vi "Common substrings.vi"(8 "minimum pattern length(3)":i32=3, 9 "Include zero transitions (t)":bool=TRUE, 11 "Full transition sequence from service to end":string[](array[string])=["-2 0 3 0 -3 0 4 -4 0\r\n", "0 3\r\n", "0 4 -3 0 -4 1 0 4 -3 0\r\n", "0\r\n", "-2 0 3 -3 0 -4 1 -4 0 3 -3 4 -3 0 2 0 3\r\n", "0 3 0 1\r\n", "0 1 0 3\r\n", "0 3 -2 0 4\r\n", "0\r\n", "0 -3 4 0 2 -2 0 -3 0 3 -2 3 -3 4\r\n", "0 -3 4 -3 0\r\n", "-2 0 -2 2 0\r\n", "0 3 -2\r\n", "0 4 -3 0 3 -2 0 -3 4 -3 0 3 -2 2 -2 0 4 0\r\n", "2 0 1 -4 0 3 0 -4 4 0 -4 4 0 2 0 4 0 -3 4 -3 0 -4 0 4\r\n", "0 4\r\n", "-2 0 -2 0 3 0\r\n", "0 3 0 -2 3\r\n", "0 4 0 4 -4 0 2 0 -4 4 -3 0 -2 2 -2 0 4 -3 0 2 0 3 0\r\n", "0 4 -3 0 1 -1 0 3 0 -2 2 -2 0 -3 4 -3 0 4 -4 1 0\r\n", "", "0 -3\r\n", "2 0 3 0 1 0 -2 3\r\n", "0\r\n", "1 -1 0\r\n", "0 -2 3 0\r\n", "0 1 0 4 0 4 -4 4\r\n", "0 1 -1 0 3\r\n", "0 2 -2 3 -3 4\r\n", "-2 2 0 -2 3\r\n", "0 -1\r\n", "0 4 -4 4 0 3 0 -2 0 -4 0 1 -4\r\n", "-2 0 4 0 -3 3 0 -2 2 -2 0 -4 0 4 0\r\n", "0 -1 0 -4 4 -4 1 -4 0\r\n", "1 -4 1 0 2 0 -3 0 2 0 -2 0 1 0 1 -4 4 -4 1 0 3 -2 0 -4 4 -4\r\n", "0 1 -4 4 -4 1\r\n", "0 3 0 -3 3 0 1 0 1 -4 4\r\n", "0 1 -4 0 1 -4\r\n", "0 3 -2 0 1 -4 1 0 2 0 4 0 4 0 -1 2 -1 0\r\n", "1 0 -1 0 2 0 4 -4\r\n", "-4\r\n", "-1 0 4\r\n", "0 1 -1 0 1 -4 0\r\n", "-1 0 1 -4 0 3 0 2 0 4 0 -4 4 -4 0 -1 0 -4 0 -2 0 4\r\n", "0 4 0\r\n", "0 4 -4 0 2 -1 0 2 0 4 -4 1 -4 4 0 3\r\n", "0 4 0 2 0\r\n", "1 0 -1 1 0 -4 1 -4 1 0 -4\r\n", "0 3 -2 0 -4\r\n", "2 -1 0 -4 4 -4 0 2 0 4\r\n", "1 0\r\n", "-1 0 -1 1 0 -4\r\n", "0 3 0\r\n", "0 -4 4 -4 0 -4 0 4 0 2 0 1 -4 4\r\n", "-1 0 1 -4\r\n", "-1 0 2 -1 0 2\r\n", "1 -1 0 4 -4 1\r\n", "-1 0 1 -4 4 -4 0 -4 4\r\n", "0 3 0 3 0 1 -1 0 1\r\n", "-1 0 4 0 4 -4 1 0 -4 0\r\n", "1 0 4\r\n", "0 -1 0 2 -1 0 -2 3 -2 0 -4 4 -4\r\n", "0 3 0\r\n", "2 -1 0 1 -4 4 -4 0 2 0\r\n", "0 4 -4 1 0 1 0 1 -4 0 2 0 4 0 4 -4 1\r\n", "1 -1 0 3 0 3 0 1 0 4\r\n", "0 -4 0 -2 0 -4\r\n", "0 -4 4 -4 0 -2 0 2 0\r\n", "-1 0 4 -4 0\r\n", "1 0 -1 2 0 4\r\n", "0 2 0 -2 0\r\n", "0 1 -4 0 -4 0 3 -2 0 -4 0 -4 4 -4 1\r\n", "0 4 0 4 0 4 0 4 0 -2 3 0 3 0 4 0\r\n", "-4 -1\r\n", "-2 0 1 0 -4 4\r\n", "0 4\r\n", "-2 2 0 -1 -4 1 0 3 0\r\n", "-1 0 -1 2\r\n", "0 -1 1 0 4 0 3 -2 0 -2 3 -2 0 4 0 -2 2\r\n", "2 -1 0 4\r\n", "0 4 0 2 0 -2 0\r\n", "1 -1 0 3 0 -4 4 -4 0\r\n", "2 -1 0 3 -2 0 -3 0 3 0 -3 0\r\n", "0 4 0 4 -4 1 -1 0 -3 0 1 -4 1 0 4 0 -4 0 -4 4 -4 1\r\n", "0 -4 1 0 -4 4\r\n", "0 4 0 -2 2 -2 2 -2 2\r\n", "-2 2 -1 0 4 0 2 0 4 0 2 -2 0 4\r\n", "1 0 -1 0 -1 0 1 -1\r\n", "-2 2 -2 3\r\n", "1 0 -1 0 -1 2 0 2 -2 0 -4 0\r\n", "-2 2 0 3 -2 2\r\n", "0\r\n", "1 -1 0 3\r\n", "0 4 0\r\n", "-2 0 1 -4 0 -3 0\r\n", "1 0 -1 2 -1 1 -4\r\n", "0 4\r\n", "-2 0 -1 1\r\n", "0 3 0 3 0 3 -2\r\n", "-4 0 -4 4\r\n", "0 4 0 -4 0 -4\r\n", "-2 2 0 4 -4 0 2 -2\r\n", "-2 2 -2 0 -1\r\n", "0 4 -3 0\r\n", "0 1 0 -1 1\r\n", "-4 0\r\n", "-2 0 3 0 1 0 3 -2 0 -1 0 4 0 3 0 -3 3 -3\r\n", "0 4 0 -2 0 1 0 -4 4 -3 0 1 0 4 0 -4 1 0 3 -3 0\r\n", "0 -1 2\r\n", "2 0 -3 4 0\r\n", "-4 0 -3 3 -3 0 -3 3 0 -2 3 0\r\n", "0 -1 1 -4 4 -3 0 3 0\r\n", "0 -1 2 0 3 0 1 -4 4 0 2 0\r\n", "2 -2 0 -4 0 -4 4 0 -4\r\n", "1 -1 2 -1\r\n", "2 0 -2 0 4 0 2 0 3 0 -2 0 -4\r\n", "1 -1 0 -1\r\n", "0 1 -4 1\r\n", "0 4 0 -1 1 -1 0\r\n", "0 3\r\n", "-2 0\r\n", "1 -4 0 -2 0 4 0 -4 0 4 -3 0 1 -4 0 1\r\n", "0 -3 3 -2 0 3 0 -2 2\r\n", "1 0\r\n", "2\r\n", "0 -4\r\n", "0 4 0 -4 0 -3 3 -3 0 -2 0 -2 0 4 0 -1 1 0 3 0 -4 1 -4 0 4\r\n", "2 0 -1 1\r\n", "0 2 0 4 0 4 -4 0 -1 2\r\n", "0 3 -2 0 3 -2\r\n", "1 0 -3 3 0 -4\r\n", "0 -3 3 0 -1 0\r\n", "2 -2 0 1\r\n", "-4 1 -4 1 -4 0\r\n", "0 4 0 2 0 -4 1 2 -1 0 4 0 1 0 4 -4 4 0 -4 4 0\r\n", "-2 0 3 0 -2 0\r\n", "-2 2 -1 0 1 -4 0 3 -2\r\n", "1 -1 0 4 0 2 -2 3 0 1 -4 1 0 -3 4 0 3 0 4 0 4 0 -4 0\r\n", "-1 0 4 -4\r\n", "-1 0 -1 2 0 2 0\r\n", "-1 0 3 -2 0 2 -2 3 -2 2 -2 0 -3 4 0 1\r\n", "-2 2 -1 0 2 0 3 -1 3 -2 2 0 -2 2 -2 0 1 0 2 0\r\n", "1 -4 1 0 4 -4 0 2 0\r\n", "2 -2 0\r\n", "0 4 -4 -1 0 -1 1 -1 0 4 0 -2 3 -2 0\r\n", "-1 0 2 -1 0 4 -4 0 -4 0 4 0\r\n", "0 -3 0\r\n", "1 0 -1 2 -1 0 3 0 3 -2 3 -2 0 2\r\n", "2 0 2 0 -2 3 -2 2 -1 0 4 0 2\r\n", "-1 1 -4 1 0 1 0 -4 4 -4 0 3 -2 2 -1 0 3 0 -1 1\r\n", "2 0 -1 1 -1 0 3 -2 3 0 2 0 3 -2 0 -4 0 4 -4 0 4 0\r\n", "0 -1 0 3 0 2 -2\r\n", "1 -4 1 -1 0 2 0 3 -2 3 -2 3\r\n", "2 0\r\n", "-1 0 3 0 3\r\n", "1 -4 1 0 -4 4 -4 0\r\n", "-2 2 -1 0\r\n", "0 1 0 4 0 3 0 -2 0 3 0 4 0 2 -2 0\r\n", "0 3 -2 0 4 0 -2 2 -2 0 -2 0 4 0 -2 0 2\r\n", "2 0 1 -1 0\r\n", "1 0 -3 4 -3 0 -2 0 3 0\r\n", "0 3 -2 0 4 0 -3 3 0 3 -2 0\r\n", "2 0 3 0 1 0 3\r\n", "1 0 3 -3 0 4 -3 0\r\n", "-2 2 -2 0\r\n", "0 1 0 -3 4 0 3 -2 3 0 1 0 4 0 -1\r\n", "0 3\r\n", "-2 2 0 3 0 -2 0 2 0 -2 0 3 0 -4 0 -2\r\n", "0 3 0 -3 4\r\n", "0 3 -2 2 -2 3 -2 0\r\n", "-1 0 3 0 3\r\n", "2 0\r\n", "0 -3 0 1\r\n", "1 0 4 -4 1\r\n", "-2 2 0 4 0 -2 0 -2\r\n", "1 0 4 0 1 0 -3 3\r\n", "-2 2 0 3 -2\r\n", "1 0 -3 4 -3 0 3 0 3 0 -2 0 3 -2 0 1 -4 0 3 0 -2 0 3 -3 0\r\n", "-2 2 0 2 0 3\r\n", "0 3 -2 0 3 0 -4 1\r\n", "0 1 0 -4 4 0 -2 0 3 0 -4 0 4 0 -4 1 0 3 -2 3 0 -1 1 -1\r\n", "2 0 -3 4 -3 0 2 0\r\n", "0 3\r\n", "0 3\r\n", "-1 0 4\r\n", "0 3\r\n", "-2 3 0 1 -4 0 -2 2 -2 3 0 4\r\n", "2 -2 0 4 0 -4 1 -4 0 3 -2\r\n", "1 0 2\r\n", "0 3 0 2 -2 3 -3 0 1 0 -3 3 0 4 0 2 -2 2 -2 3 0\r\n", "2 0 -2 3 2\r\n", "0 1 0 4 -4 1 -1 2 -2 3 -3 0 -2\r\n", "0 -3 4 -3 0 2\r\n", "0 2 -2 3\r\n", "0 -4 0 -4 1 0 3 0 1 0 2 -2 0 -3 4 0 4 -3 0 3 -3 -2 0 -3 4 0 -4 0 3 0\r\n", "-2 2 -2 3 -3 0 -4 1\r\n", "0 -2 0 2 0 4 0\r\n", "0 -3 0 -4 0 -3 4 0 -2 3 -3\r\n", "2 0 -2 2 0 4 0 1 0 -2 3\r\n", "0 4 0 3 -2 3 0 -4 4 0 4 0 3 0 3\r\n", "2 0 -2 0 4 0 3 -2 2 -2 3 0 -2\r\n", "1 0 3 -3 0 3 0 3 -2 3 -2 3 0 3 0 -1 0 4 0 -4 1 0 3\r\n", "2 -2 0 -3 4 -3\r\n", "0 1 0 3 0 -2 2 -2\r\n", "1 0\r\n", "2 0 -2 3 -2 2 0\r\n", "1 0 -4 4 0 3 -2 3 -2 0 4 -3 0 -3 4 0 -4 1 -4 0 2 -2 0 3 -3 0 1 0 3 0 -2 3 0 4 0 -4 1 0 3 0 -3 4 0 2\r\n", "0 -3 4 -3 0 1 0\r\n", "0 3 0 4 0 -4 1 0 -2 0\r\n", "2 -2 0 -2 0 -4\r\n", "-1 0\r\n", "2 0 4\r\n", "1 0 3 0\r\n", "2 0 -4 4 0 1 0 3 -2 0 4 0 -4 0 3 0 -2 3\r\n", "0 2 -2 0 -4 0 -4 4 -3 0 -4 1 0 4 0 -3 3 0\r\n", "1 0 4 -3 0 2 -2 0 4 0 -3 4 -3 0 -4 0 -3 0 -4 1 0 -2 3 -2 0 1\r\n", "2 -2 3 0\r\n", "2 -1 0 4 0 1 0 3 -2\r\n", "0 3 0 -2 3 -2 0 -2 3 -2 2 -1 0 3 0\r\n", "1 0 1 0 4 -4 0 3 0 3 -2 0 4 0 3 -2\r\n", "0 3 -2 0 -1 1 0 2 -2 2 0 -3 4\r\n", "2 0 4\r\n", "0 -4 4 -4 0 1 -1 0 4\r\n", "-1 0 4 -4 0 -4 4 -4 0 2 0 -4 0 -3 3 -2 3 -2 0 -4\r\n", "2 0 -1 2 -1 0 1 -1 0 3 0 -2 0 3 0 -3 0 -3 0 -4 4 -4 1 -1 2 -1 1 0 3 0\r\n", "0 3\r\n", "1 0 -3 0 1 -4 0 2 0 -2 3 0 4 -4 0 -1 0 3 0 1\r\n", "0 -1 2 0 -3 4 0 -1 0 4 -4 4 -4 0 2 -1 1 0 -3 3 0\r\n", "0 3 -2 3 0 4 0 1 0 4 0 -4 4 -4 0 -4 4 -4 0 3\r\n", "2 0 3 0 1 0\r\n", "1 0 -4 1 -1 0 -2 -1 3 -2 2 -2 0 -3 0 1 -1\r\n", "2 0 3\r\n", "-4 1 -1 0 3 0 3 0 1\r\n", "0 4 0 -4 1 0 1 0 3 0 4 -4 0 -4 4 0\r\n", "2 0 -4 4 0 -1\r\n", "0 3 -2 2\r\n", "0 4 0 1 -4 4 -4 0 2 0 -3 4 0 4 -4 0 3 0 -1 1 -4 4 0 1\r\n", "0 1 -1 0 -4 0 4 0 1 0 4 0 2 0 -4 4 0 2 0 3 0 4 -4 0 3 0 4 0 -4 4\r\n", "1 0 -4 4 0 2 -1 0\r\n", "2 0 4 -4 1 -1 0 4 0 -2 2 0 4 -4 0 1 0 4 0 2\r\n", "0 4 0 3 -2 0 4\r\n", "0 3 0 -2 3 0 1 -4\r\n", "1 -4 1 0 -1 0 3 -2 2 0\r\n", "2 0 -1 0 3\r\n", "0 -1 0 2 0 -3 4 -4 0 3 0 1 -1 0 -4 4 -4 0 2 -1 1 0 3 0 4 -4 0 3 0 1 0 3 -2\r\n", "2 -1 0 3 0 4 -4 0 1 -4 1 -1 0 -4 4 0 -4 0 3 -2 0 4 -4 4 -4 0 2 -2 0 1 0 4 0 3 0 3 -2 3 -3 0 3 0 -3 0 1 -4\r\n", "1 -1 0 -2 3 -3 0 -4 0 -3 0 3 -2 0 3 -2 2\r\n", "0 4\r\n", "2 0 -2 3 0 2 -1 0 -3 0 -2 3\r\n", "1 0 3 0 3 0 -2 3 -2 0 -2 3 -2 0 3 0 1 -1 0 3 0 3 0 4 -4 0 1 -1 0 3 0 -3 0 -4 4 -4 0 3 0 -1 1 -4 1\r\n", "0 -1 2 0 3\r\n", "2 0 3 -2 0\r\n"]) -> (0 "List of common substrings and the number of times they occur":string[][](array[string]), 1 "unique substirings without repetitions":string[][](array[string]), 2 "Full patterns with common substrings to a pattern (pattern, list of main patterns)":string[][](array[string]), 3 "common substrings of a pattern with all other patterns (pattern, All substrings)":string[][](array[string]))   [LabVIEW 2013]
panel:
  out "Numeric 2":i32
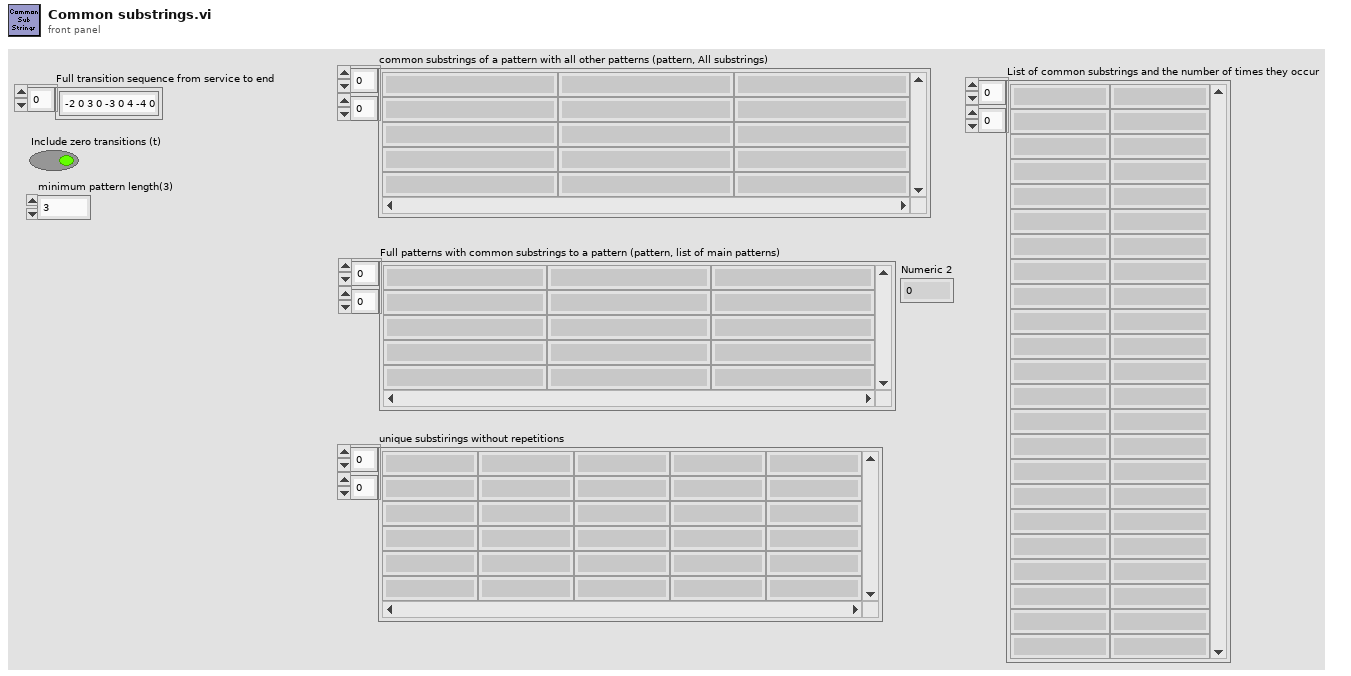
[diagram p1: front panel]
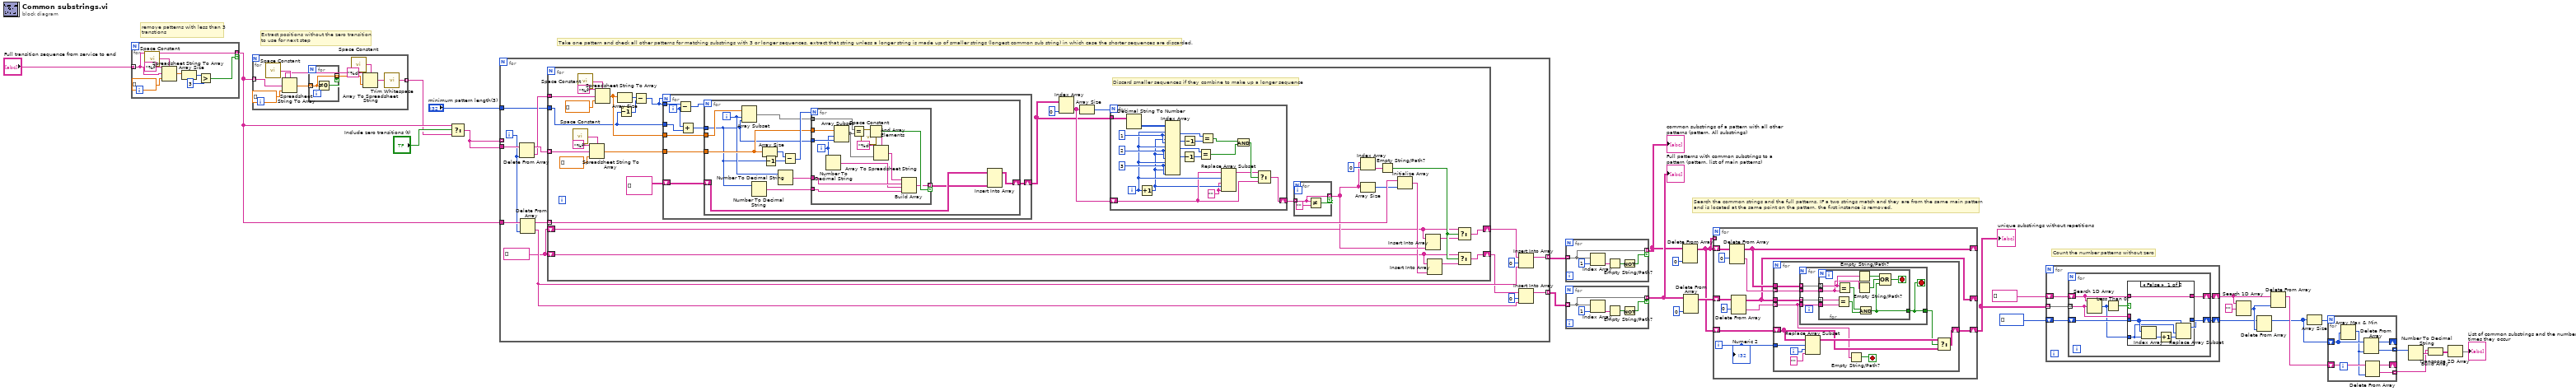
[diagram p0: block diagram]
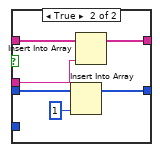
[diagram p2: hidden frame]
diagram:
  # "Count the number patterns without zero"
  # "Search the common strings and the full patterns. IF a two strings match and they are from the same main pattern\nand is located at the same point on the pattern, the first instance is removed."
  # "Extract positions without the zero transition\nto use for next step"
  # "remove patterns with less than 3\ntranstions"
  # "Take one pattern and check all other patterns for matching substrings with 3 or longer sequences. extract that string unless a longer string is made up of smaller strings (longest common sub string) in which case the shorter sequences are discarded."
  n1 = for {
    tunnel: "Full transition sequence from service to end" -> [w31] mode=indexing
    tunnel: [w31] -> w4 mode=indexing if=w30
    n2 = call <vilib>:"Space Constant.vi"() -> ("String"=w36:string)
    n3 = Spreadsheet String To Array(delimiter (Tab)=w36, format string="%f", spreadsheet string=w31, array type (2D Dbl)=dbl[] [] ("array 2")) -> (array=w34:dbl[])
    n4 = Array Size(array=w34) -> (size(s)=w33:i32)
    n5 = Greater?(x=w33, y=3) -> (0:w30:bool)
  }
  n6 = for {
    tunnel: w4 -> [w44] mode=indexing
    tunnel: [w38] -> w3 mode=indexing
    w41 = "%d" ("format string")
    n7 = call <vilib>:"Space Constant.vi"() -> ("String"=w46:string)
    n8 = Spreadsheet String To Array(delimiter (Tab)=w46, format string=w41, spreadsheet string=w44, array type (2D Dbl)=dbl[] [] ("array 2")) -> (array=w43:dbl[])
    n9 = for {
      tunnel: w43 -> [w48] mode=indexing
      tunnel: [w48] -> w42 mode=indexing if=w47
      n10 = Not Equal To 0?(x=w48) -> (x != 0?=w47:bool)
    }
    n11 = call <vilib>:"Space Constant.vi"() -> ("String"=w40:string)
    n12 = Array To Spreadsheet String(delimiter (Tab)=w40, array=w42, 3:w41) -> (spreadsheet string=w39:string)
    n13 = call <vilib>:"Trim Whitespace.vi"("string"=w39) -> ("trimmed string"=w38:string)  [unwired: 1 in]
  }
  n14 = Select(t=w4, s="Include zero transitions (t)", f=w3) -> (s? t:f=w6:string[])
  n15 = for {
    tunnel: w6 -> [_] mode=indexing
    tunnel: w6 -> [w63]
    tunnel: [w60] -> w29 mode=indexing
    tunnel: w4 -> [w59]
    tunnel: [w53] -> w28 mode=indexing
    tunnel: "minimum pattern length(3)" -> [w49]
    i -> [w58]
    w52 = string[] []
    n16 = Delete From Array(array=w63, index=w58) -> (deleted portion=w57:string, array with subset deleted=w62:string[])  [unwired: 1 in]
    n17 = Delete From Array(array=w59, index=w58) -> (deleted portion=w54:string, array with subset deleted=w56:string[])  [unwired: 1 in]
    n18 = for {
      tunnel: w62 -> [w78] mode=indexing
      tunnel: w57 -> [w79]
      tunnel: w56 -> [w76] mode=indexing
      shift-right: [w66] -> w50
      shift-left: w52 -> [w70]
      shift-right: [w68] -> w51
      shift-left: w52 -> [w71]
      tunnel: w49 -> [w64]
      # "Discard smaller sequences if they combine to make up a longer sequence"
      n19 = call <vilib>:"Space Constant.vi"() -> ("String"=w84:string)
      n20 = call <vilib>:"Space Constant.vi"() -> ("String"=w81:string)
      n21 = Spreadsheet String To Array(delimiter (Tab)=w84, format string="%f", spreadsheet string=w78, array type (2D Dbl)=dbl[] [] ("array 2")) -> (array=w88:dbl[])
      n22 = Spreadsheet String To Array(delimiter (Tab)=w81, format string="%f", spreadsheet string=w79, array type (2D Dbl)=dbl[] [] ("array 2")) -> (array=w87:dbl[])
      n23 = Array Size(array=w87) -> (size(s)=w86:i32)
      n24 = Decrement(x=w64) -> (x-1=w65:i32)
      n25 = Subtract(x=w86, y=w65) -> (x-y=w90:i32)
      n26 = for {
        N: w90 -> [_]
        tunnel: w90 -> [w128]
        tunnel: w87 -> [w124]
        tunnel: w88 -> [w123]
        shift-right: [w121] -> w77
        shift-left: string[][] [] -> [w122]
        tunnel: w64 -> [w120]
        i -> [w126]
        n27 = Subtract(x=w128, y=w126) -> (x-y=w127:i32)
        n28 = Add(x=w126, y=w120) -> (x+y=w125:i32)
        n29 = for {
          N: w127 -> [_]
          tunnel: w125 -> [w129]
          tunnel: w124 -> [w141]
          tunnel: w123 -> [w137]
          shift-right: [w134] -> w121
          shift-left: w122 -> [w135]
          i -> [w133]
          n30 = Array Subset(array=w141, index=w133, length=w129) -> (w136:dbl[])
          n31 = Number To Decimal String(number=w129) -> (decimal integer string=w131:string)  [unwired: 1 in]
          n32 = Array Size(array=w137) -> (size(s)=w140:i32)
          n33 = Decrement(x=w129) -> (x-1=w139:i32)
          n34 = Number To Decimal String(number=w133) -> (decimal integer string=w132:string)  [unwired: 1 in]
          n35 = Subtract(x=w140, y=w139) -> (x-y=w138:i32)
          n36 = for {
            N: w138 -> [_]
            tunnel: w137 -> [w155]
            tunnel: w129 -> [w154]
            tunnel: w136 -> [w153]
            tunnel: [w145] -> w130 mode=indexing if=w148
            tunnel: w132 -> [w146]
            tunnel: w131 -> [w142]
            i -> [w144]
            n37 = Number To Decimal String(number=w144) -> (decimal integer string=w143:string)  [unwired: 1 in]
            n38 = Array Subset(array=w155, index=w144, length=w154) -> (w149:dbl[])
            n39 = Equal?(x=w153, y=w149) -> (x = y?=w152:bool[])
            n40 = call <vilib>:"Space Constant.vi"() -> ("String"=w151:string)
            n41 = And Array Elements(Boolean array=w152) -> (logical AND=w148:bool)
            n42 = Array To Spreadsheet String(delimiter (Tab)=w151, array=w149, 3:"%d" ("format string")) -> (spreadsheet string=w147:string)
            n43 = Build Array(w147, w146, w143, w142) -> (w145:string[])
          }
          n44 = Insert Into Array(array=w135, new element=w130) -> (w134:string[][])  [unwired: 2 in]
        }
      }
      n45 = Index Array(array=w77, index (col)=0 ("disabled index (col)")) -> (element=w92:string[])  [unwired: 1 in]
      n46 = Array Size(array=w92) -> (size(s)=w91:i32)
      n47 = for {
        N: w91 -> [_]
        tunnel: w77 -> [w116]
        shift-right: [w102] -> w94
        shift-left: w92 -> [w103]
        i -> [w106]
        w100 = "" ("new element/subarray")
        w117 = 3 ("index (col)")
        w118 = 2 ("index (col)")
        w119 = 1 ("disabled index (col)")
        n48 = Decimal String To Number(string=w116) -> (number=w115:i32[][])  [unwired: 2 in, 1 out]
        n49 = Increment(x=w106) -> (x+1=w101:i32)
        n50 = Index Array(array=w115, index (row) #1=w106, index (col) #1=w119, index (row) #2=w101, index (col) #2=w119, index (row) #3=w106, index (col) #3=w118, index (row) #4=w101, index (col) #4=w118, index (row) #5=w106, index (col) #5=w117, index (row) #6=w101, index (col) #6=w117) -> (element #1=w110:i32, element #2=w114:i32, element #3=w109:i32, element #4=w113:i32)  [unwired: 2 out]
        n51 = Decrement(x=w113) -> (x-1=w111:i32)
        n52 = Decrement(x=w114) -> (x-1=w112:i32)
        n53 = Equal?(x=w109, y=w111) -> (x = y?=w108:bool)
        n54 = Equal?(x=w110, y=w112) -> (x = y?=w107:bool)
        n55 = Replace Array Subset(array=w103, new element #1=w100, index #1=w106, new element #2=w100, index #2=w101) -> (w104:string[])
        n56 = And(x=w107, y=w108) -> (x .and. y?=w105:bool)
        n57 = Select(t=w104, s=w105, f=w103) -> (s? t:f=w102:string[])
      }
      n58 = for {
        tunnel: w94 -> [w98] mode=indexing
        tunnel: [w98] -> w74 mode=indexing if=w97
        n59 = Not Equal?(x=w98, y="") -> (x != y?=w97:bool)
      }
      n60 = Array Size(array=w74) -> (size(s)=w75:i32)
      n61 = Index Array(array=w74, index=0) -> (element=w95:string)
      n62 = Empty String/Path?(string/path=w95) -> (empty?=w72:bool)
      n63 = Initialize Array(w76, w75) -> (w73:string[])
      n64 = Insert Into Array(array=w70, new element=w74) -> (w67:string[])  [unwired: 1 in]
      n65 = Insert Into Array(array=w71, new element=w73) -> (w69:string[])  [unwired: 1 in]
      n66 = Select(t=w70, s=w72, f=w67) -> (s? t:f=w66:string[])
      n67 = Select(t=w71, s=w72, f=w69) -> (s? t:f=w68:string[])
    }
    n68 = Insert Into Array(array=w50, index=0, new element=w54) -> (w60:string[])
    n69 = Insert Into Array(array=w51, index=0, new element=w54) -> (w53:string[])
  }
  n70 = for {
    tunnel: w29 -> [w157] mode=indexing
    tunnel: [w157] -> w7 mode=indexing if=w156
    n71 = Index Array(array=w157, index=1) -> (element=w159:string)
    n72 = Empty String/Path?(string/path=w159) -> (empty?=w158:bool)
    n73 = Not(x=w158) -> (.not. x?=w156:bool)
  }
  "common substrings of a pattern with all other patterns (pattern, All substrings)" <- w7
  n74 = for {
    tunnel: w28 -> [w162] mode=indexing
    tunnel: [w162] -> w8 mode=indexing if=w161
    n75 = Index Array(array=w162, index=1) -> (element=w164:string)
    n76 = Empty String/Path?(string/path=w164) -> (empty?=w163:bool)
    n77 = Not(x=w163) -> (.not. x?=w161:bool)
  }
  "Full patterns with common substrings to a pattern (pattern, list of main patterns)" <- w8
  n78 = Delete From Array(array=w7, index (col)=0 ("disabled index (col)")) -> (array with subset deleted=w24:string[][])  [unwired: 2 in, 1 out]
  n79 = Delete From Array(array=w8, index (col)=0 ("disabled index (col)")) -> (array with subset deleted=w25:string[][])  [unwired: 2 in, 1 out]
  n80 = for {
    tunnel: w24 -> [_] mode=indexing
    shift-right: [w174] -> _
    shift-left: w24 -> [w176]
    shift-right: [w172] -> w26
    shift-left: w24 -> [w173]
    shift-right: [w166] -> _
    shift-left: w25 -> [w171]
    i -> [w169]
    n81 = Delete From Array(array=w176, index (row)=0) -> (deleted portion=w175:string[], array with subset deleted=w174:string[][])  [unwired: 2 in]
    n82 = Delete From Array(array=w171, index (row)=0) -> (deleted portion=w170:string[], array with subset deleted=w166:string[][])  [unwired: 2 in]
    n83 = for {
      tunnel: w175 -> [w187] mode=indexing
      tunnel: w174 -> [w188]
      tunnel: w169 -> [w186]
      shift-right: [w181] -> w172
      shift-left: w173 -> [w182]
      tunnel: w166 -> [w180]
      tunnel: w170 -> [w177] mode=indexing
      i -> [w185]
      stop <- w178 stop-if-true
      n84 = for {
        tunnel: w188 -> [w193] mode=indexing
        tunnel: w187 -> [w192]
        tunnel: [w189] -> w179
        tunnel: w177 -> [w191]
        tunnel: w180 -> [w190] mode=indexing
        stop <- w189 stop-if-true
        n85 = for {
          tunnel: w193 -> [w199] mode=indexing
          tunnel: w192 -> [w198]
          tunnel: w191 -> [w202]
          tunnel: w190 -> [w203] mode=indexing
          tunnel: [w195] -> w189
          stop <- w194 stop-if-true
          n86 = Equal?(x=w203, y=w202) -> (x = y?=w201:bool)
          n87 = Equal?(x=w199, y=w198) -> (x = y?=w200:bool)
          n88 = Empty String/Path?(string/path=w199) -> (empty?=w197:bool)
          n89 = Empty String/Path?(string/path=w198) -> (empty?=w196:bool)
          n90 = And(x=w200, y=w201) -> (x .and. y?=w195:bool)
          n91 = Compound Arithmetic op=OR(w197, w196, w195) -> (w194:bool)
        }
      }
      n92 = Replace Array Subset(array=w182, new element="" ("new element/subarray"), index (row)=w186, index (col)=w185) -> (w183:string[][])
      n93 = Empty String/Path?(string/path=w177) -> (empty?=w178:bool)
      n94 = Select(t=w183, s=w179, f=w182) -> (s? t:f=w181:string[][])
    }
    "Numeric 2" <- w169
  }
  "unique substirings without repetitions" <- w26
  n95 = for {
    tunnel: w26 -> [w208] mode=indexing
    shift-right: [w207] -> w14
    shift-left: string[] [] -> [w206]
    shift-right: [w204] -> w15
    shift-left: i32[] [] -> [w205]
    n96 = for {
      tunnel: w208 -> [w212] mode=indexing
      shift-right: [w214] -> w207
      shift-left: w206 -> [w215]
      shift-right: [w210] -> w204
      shift-left: w205 -> [w211]
      n97 = Search 1D Array(1D array=w215, element=w212) -> (index of element=w209:i32)  [unwired: 1 in]
      n98 = Less Than 0?(x=w209) -> (x < 0?=w213:bool)
      n99 = case shown="False" w213 {
        tunnel: w215 -> [w221 w227]
        tunnel: w212 -> [_ w226]
        tunnel: [w221 w225] -> w214
        tunnel: w211 -> [w219 w224]
        tunnel: w209 -> [w217 _]
        tunnel: [w216 w223] -> w210
        frame False {
          n100 = Index Array(array=w219, index=w217) -> (element=w218:i32)
          n101 = Increment(x=w218) -> (x+1=w220:i32)
          n102 = Replace Array Subset(array=w219, new element=w220, index=w217) -> (w216:i32[])
        }
        frame True {
          n103 = Insert Into Array(array=w224, new element=1 ("new element/subarray")) -> (w223:i32[])  [unwired: 1 in]
          n104 = Insert Into Array(array=w227, new element=w226) -> (w225:string[])  [unwired: 1 in]
        }
      }
    }
  }
  n105 = Search 1D Array(1D array=w14, element="") -> (index of element=w16:i32)  [unwired: 1 in]
  n106 = Delete From Array(array=w15, index=w16) -> (array with subset deleted=w18:i32[])  [unwired: 1 in, 1 out]
  n107 = Delete From Array(array=w14, index=w16) -> (array with subset deleted=w19:string[])  [unwired: 1 in, 1 out]
  n108 = Array Size(array=w18) -> (size(s)=w17:i32)
  n109 = for {
    N: w17 -> [_]
    shift-right: [w233] -> _
    shift-left: w18 -> [w234]
    tunnel: [w232] -> w20 mode=indexing
    shift-right: [w229] -> _
    shift-left: w19 -> [w231]
    tunnel: [w228] -> w21 mode=indexing
    n110 = Array Max & Min(array=w234) -> (max index (indices)=w230:i32)  [unwired: 3 out]
    n111 = Delete From Array(array=w234, index=w230) -> (deleted portion=w232:i32, array with subset deleted=w233:i32[])  [unwired: 1 in]
    n112 = Delete From Array(array=w231, index=w230) -> (deleted portion=w228:string, array with subset deleted=w229:string[])  [unwired: 1 in]
  }
  n113 = Number To Decimal String(number=w20) -> (decimal integer string=w22:string[])  [unwired: 1 in]
  n114 = Build Array(w21, w22) -> (w23:string[][])
  n115 = Transpose 2D Array(2D array=w23) -> (transposed array=→"List of common substrings and the number of times they occur":string[][])
